vi "Main Voice.vi"() -> ()   [LabVIEW 2017]
uses:
  <vilib>/MakerHub/LINX/Public/Peripherals/Digital/Digital Write 1 Chan.vi
  <vilib>/MakerHub/LINX/Public/Peripherals/Digital/Digital Write N Chans.vi
  <vilib>/MakerHub/LINX/Private/Local IO/LinxDigitalWrite.vi
  <vilib>/MakerHub/LINX/Public/Utilities/Check Channel.vi
  <vilib>/MakerHub/LINX/Public/Utilities/Open Serial.vi
  <vilib>/MakerHub/LINX/Private/Utilties/Generate Error.vi
  <vilib>/MakerHub/LINX/LMH-LINX.lvlib
panel:
  out "Command":string
  in  "Error In":errorcluster
  out "Error Out":errorcluster
  in  "Exit":bool
  out "Voice Command":string
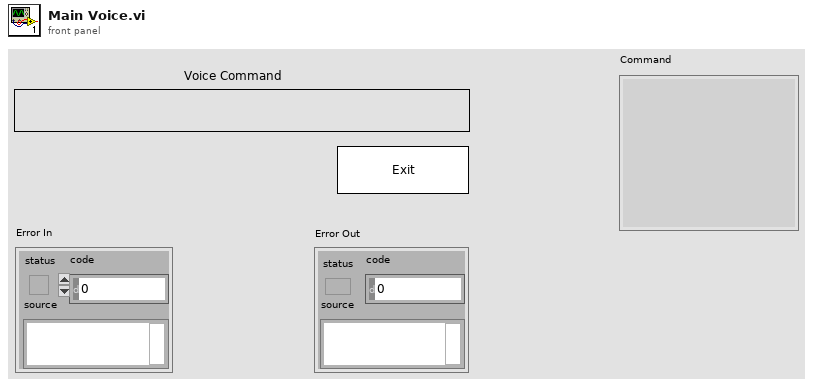
[diagram p1: front panel]
types:
  T1 = typedef "LMH-LINX.lvlib/LINX Ref.ctl" = cluster{"IO":T2, "Interface":T3, "LINX Device Config":T4}
  T2 = typedef "LMH-LINX.lvlib/Platform.ctl" = enum16{"Remote", "Local"}
  T3 = typedef "LMH-LINX.lvlib/Interface.ctl" = enum16{"Serial", "TCP"}
  T4 = typedef "LMH-LINX.lvlib/Device.lvlib/LINX Device Config.ctl" = cluster{"Interface":T3, "COM Port":refnum<visa-resource-name>, "TCP Configuration":T5, "Device Family":u8, "Device ID":u8, "Device Name":string, "TCP Ref":refnum<k5>, "Channels":T6}
  T5 = typedef "LMH-LINX.lvlib/Device.lvlib/TCP Config.ctl" = cluster{"IP Address":string, "Port":u16}
  T6 = typedef "LMH-LINX.lvlib/Channels.ctl" = cluster{"DI":u8[], "DO":u8[], "AI":u8[], "AO":u8[], "PWM":u8[], "QE":u8[], "UART":u8[], "I2C 2":u8[], "SPI":u8[], "CAN":u8[], "Servo":u8[], "AI Ref (V)":dbl, "AI Resolution (Bits)":u8, "AO Ref (V)":dbl, "AO Resolution (Bits)":u8}
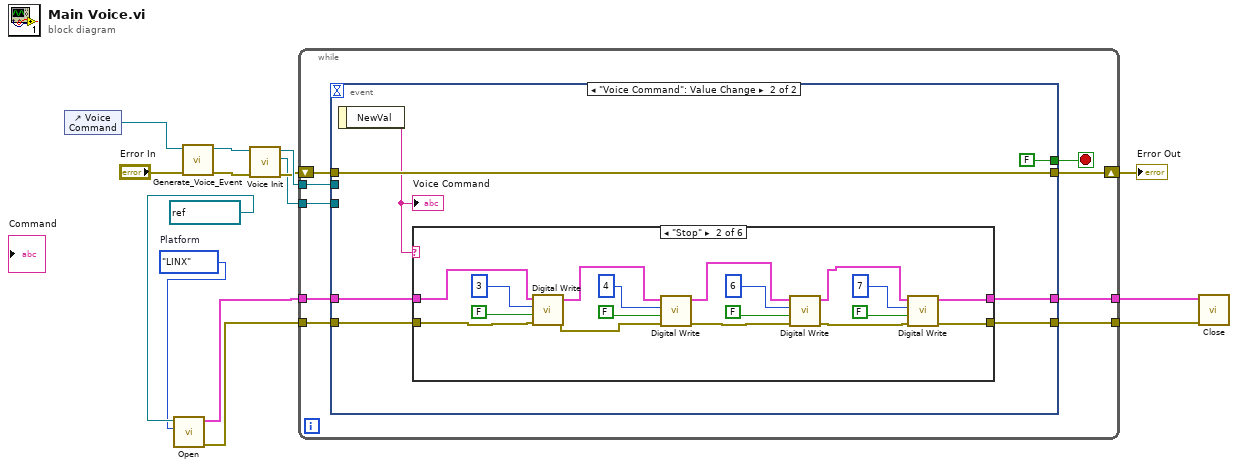
[diagram p0: block diagram]
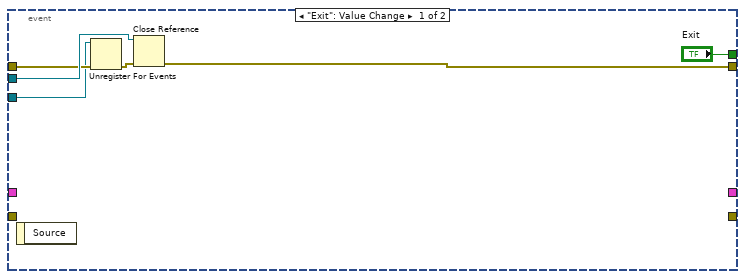
[diagram p2: hidden frame]
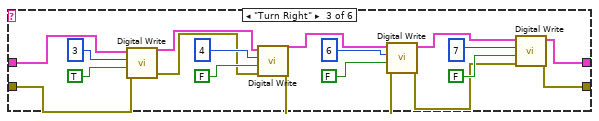
[diagram p4: hidden frame]
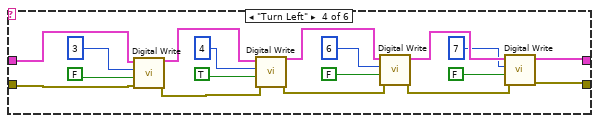
[diagram p5: hidden frame]
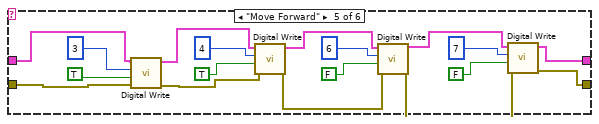
[diagram p6: hidden frame]
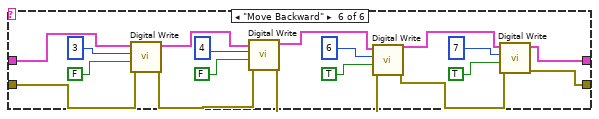
[diagram p7: hidden frame]
diagram:
  w1 = enum16{"Default", "LINX", "myRIO"}."LINX"  # Platform
  n1 = control-ref of="Voice Command"() -> (w13:refnum<vi>)
  n2 = call-poly <vilib>:"Open.vi"("Baud Rate Override"=w1, "Serial Port"=refnum<visa-resource-name> "COM9") -> ("Error Out"=w4:errorcluster, "LINX Resource"=w5:T1)  [unwired: 7 in, 1 out]
  n3 = call "Generate_Voice_Event.vi"("Error In"="Error In", "String in"=w13) -> ("Error Out"=w12:errorcluster, "String out"=w14:refnum<vi>)  [unwired: 8 in]
  n4 = call "Voice Init.vi"("Error In"=w12, "Text"=w14) -> ("Error Out"=w10:errorcluster, "Event Callback"=w7:refnum<k27>, "Reference"=w11:refnum<k24>)  [unwired: 7 in]
  n5 = while {
    tunnel: w11 -> [w22]
    shift-right: [w20] -> w9
    shift-left: w10 -> [w21]
    tunnel: w7 -> [w19]
    tunnel: w5 -> [w18]
    tunnel: w4 -> [w17]
    tunnel: [w16] -> w3
    tunnel: [w15] -> w2
    stop <- w23 stop-if-true
    n6 = event shown="[1] \"Voice Command\": Value Change" {
      selector: _ -> [_ _]
      dyn-events: _ -> [_ _]
      timeout: _ -> [_ _]
      tunnel: ["Exit" FALSE ("Exit")] -> w23
      tunnel: w22 -> [w28 _]
      tunnel: w21 -> [w26 w36]
      tunnel: [w25 w36] -> w20
      tunnel: w19 -> [w24 _]
      tunnel: w18 -> [_ w33]
      tunnel: w17 -> [_ w32]
      tunnel: [_ w31] -> w16
      tunnel: [_ w30] -> w15
      event "Exit": Value Change {
        n7 = event-data() -> ()  [unwired: 1 in, 1 out]
        n8 = Unregister For Events(event registration refnum=w24, error in=w26) -> (error out=w27:errorcluster)
        n9 = Close Reference(reference=w28, error in (no error)=w27) -> (error out=w25:errorcluster)
      }
      event "Voice Command": Value Change {
        n10 = event-data() -> ("NewVal"=w34:string)  [unwired: 1 in]
        "Voice Command" <- w34
        n11 = case shown="\"Stop\"" w34 {
          tunnel: w33 -> [w38 w56 w74 w92 w110 w128]
          tunnel: w32 -> [w37 w53 w71 w89 w107 w125]
          tunnel: [w38 w44 w58 w76 w94 w112] -> w31
          tunnel: [w37 w43 w57 w75 w93 w111] -> w30
          frame Default {
          }
          frame "Stop" {
            n12 = call-poly <vilib>:"Digital Write.vi"("Error In"=w53, "Output Value"=FALSE, "DO Channel"=u8 3, "LINX Resource"=w56) -> ("Error Out"=w49:errorcluster, "LINX Resource"=w52:T1)  [unwired: 6 in]
            n13 = call-poly <vilib>:"Digital Write.vi"("Error In"=w49, "Output Value"=FALSE, "DO Channel"=u8 4, "LINX Resource"=w52) -> ("Error Out"=w47:errorcluster, "LINX Resource"=w48:T1)  [unwired: 6 in]
            n14 = call-poly <vilib>:"Digital Write.vi"("Error In"=w47, "Output Value"=FALSE, "DO Channel"=u8 6, "LINX Resource"=w48) -> ("Error Out"=w39:errorcluster, "LINX Resource"=w42:T1)  [unwired: 6 in]
            n15 = call-poly <vilib>:"Digital Write.vi"("Error In"=w39, "Output Value"=FALSE, "DO Channel"=u8 7, "LINX Resource"=w42) -> ("Error Out"=w43:errorcluster, "LINX Resource"=w44:T1)  [unwired: 6 in]
          }
          frame "Turn Right" {
            n16 = call-poly <vilib>:"Digital Write.vi"("Error In"=w71, "Output Value"=TRUE, "DO Channel"=u8 3, "LINX Resource"=w74) -> ("Error Out"=w67:errorcluster, "LINX Resource"=w70:T1)  [unwired: 6 in]
            n17 = call-poly <vilib>:"Digital Write.vi"("Error In"=w67, "Output Value"=FALSE, "DO Channel"=u8 4, "LINX Resource"=w70) -> ("Error Out"=w63:errorcluster, "LINX Resource"=w66:T1)  [unwired: 6 in]
            n18 = call-poly <vilib>:"Digital Write.vi"("Error In"=w63, "Output Value"=FALSE, "DO Channel"=u8 6, "LINX Resource"=w66) -> ("Error Out"=w59:errorcluster, "LINX Resource"=w62:T1)  [unwired: 6 in]
            n19 = call-poly <vilib>:"Digital Write.vi"("Error In"=w59, "Output Value"=FALSE, "DO Channel"=u8 7, "LINX Resource"=w62) -> ("Error Out"=w57:errorcluster, "LINX Resource"=w58:T1)  [unwired: 6 in]
          }
          frame "Turn Left" {
            n20 = call-poly <vilib>:"Digital Write.vi"("Error In"=w89, "Output Value"=FALSE, "DO Channel"=u8 3, "LINX Resource"=w92) -> ("Error Out"=w85:errorcluster, "LINX Resource"=w88:T1)  [unwired: 6 in]
            n21 = call-poly <vilib>:"Digital Write.vi"("Error In"=w85, "Output Value"=TRUE, "DO Channel"=u8 4, "LINX Resource"=w88) -> ("Error Out"=w83:errorcluster, "LINX Resource"=w84:T1)  [unwired: 6 in]
            n22 = call-poly <vilib>:"Digital Write.vi"("Error In"=w83, "Output Value"=FALSE, "DO Channel"=u8 6, "LINX Resource"=w84) -> ("Error Out"=w77:errorcluster, "LINX Resource"=w80:T1)  [unwired: 6 in]
            n23 = call-poly <vilib>:"Digital Write.vi"("Error In"=w77, "Output Value"=FALSE, "DO Channel"=u8 7, "LINX Resource"=w80) -> ("Error Out"=w75:errorcluster, "LINX Resource"=w76:T1)  [unwired: 6 in]
          }
          frame "Move Forward" {
            n24 = call-poly <vilib>:"Digital Write.vi"("Error In"=w107, "Output Value"=TRUE, "DO Channel"=u8 3, "LINX Resource"=w110) -> ("Error Out"=w103:errorcluster, "LINX Resource"=w106:T1)  [unwired: 6 in]
            n25 = call-poly <vilib>:"Digital Write.vi"("Error In"=w103, "Output Value"=TRUE, "DO Channel"=u8 4, "LINX Resource"=w106) -> ("Error Out"=w99:errorcluster, "LINX Resource"=w102:T1)  [unwired: 6 in]
            n26 = call-poly <vilib>:"Digital Write.vi"("Error In"=w99, "Output Value"=FALSE, "DO Channel"=u8 6, "LINX Resource"=w102) -> ("Error Out"=w95:errorcluster, "LINX Resource"=w98:T1)  [unwired: 6 in]
            n27 = call-poly <vilib>:"Digital Write.vi"("Error In"=w95, "Output Value"=FALSE, "DO Channel"=u8 7, "LINX Resource"=w98) -> ("Error Out"=w93:errorcluster, "LINX Resource"=w94:T1)  [unwired: 6 in]
          }
          frame "Move Backward" {
            n28 = call-poly <vilib>:"Digital Write.vi"("Error In"=w125, "Output Value"=FALSE, "DO Channel"=u8 3, "LINX Resource"=w128) -> ("Error Out"=w121:errorcluster, "LINX Resource"=w124:T1)  [unwired: 6 in]
            n29 = call-poly <vilib>:"Digital Write.vi"("Error In"=w121, "Output Value"=FALSE, "DO Channel"=u8 4, "LINX Resource"=w124) -> ("Error Out"=w117:errorcluster, "LINX Resource"=w120:T1)  [unwired: 6 in]
            n30 = call-poly <vilib>:"Digital Write.vi"("Error In"=w117, "Output Value"=TRUE, "DO Channel"=u8 6, "LINX Resource"=w120) -> ("Error Out"=w113:errorcluster, "LINX Resource"=w116:T1)  [unwired: 6 in]
            n31 = call-poly <vilib>:"Digital Write.vi"("Error In"=w113, "Output Value"=TRUE, "DO Channel"=u8 7, "LINX Resource"=w116) -> ("Error Out"=w111:errorcluster, "LINX Resource"=w112:T1)  [unwired: 6 in]
          }
        }
      }
    }
  }
  "Error Out" <- w9
  n32 = call <vilib>:"Close.vi"("Error In"=w2, "LINX Resource"=w3) -> ()  [unwired: 9 in, 1 out]
